vi "to string.vi"(8 "error in":errorcluster, 11 "EthernetIP configuration in":refnum<class "EthernetIP configuration.lvclass">) -> (0 "error out":errorcluster, 1 "data":string, 2 "version":string, 3 "EthernetIP configuration out":refnum<class "EthernetIP configuration.lvclass">)   [LabVIEW 2013, in "EthernetIP configuration.lvclass"]
doc: "Provides an interface for saving a module configuration to a file or other serialized data source. It is recommended that all children of this class store data in two sets--data required for its own initialization, and any data required for parent initialization--and that each implementation uses the <b>Call Parent Method</b> primitive to serialize parent information."
uses:
  EthernetIP configuration.lvclass
  <vilib>/NI/Tag Bus Module Framework/module configuration/TBM module configuration.lvclass
  EthernetIP configuration.lvclass/EthernetIP configuration.ctl
  <vilib>/NI/Tag Bus Module Framework/root configuration/unwrap data.vi
  <vilib>/NI/Tag Bus Module Framework/root configuration/TBM configuration.lvclass
  channel/EthernetIP Channel.lvclass
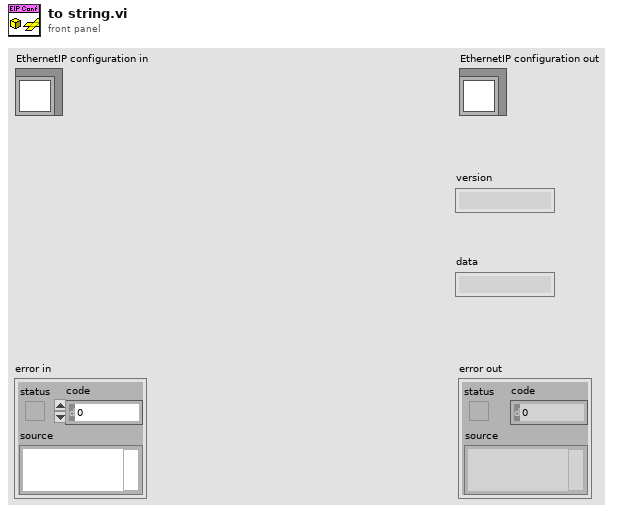
[diagram p1: front panel]
types:
  T1 = typedef "EthernetIP configuration.lvclass/assembly definition.ctl" = cluster{"name":string, "Instance ID":u32, "Type":T2, "Size (elements)":u32, "big endian?":bool, "data type":T3}
  T2 = typedef "EthernetIP configuration.lvclass/assembly type.ctl" = enum32{"Producing", "Consuming"}
  T3 = typedef "tag bus.lvlib/tag descriptor.lvclass/Data Type.ctl" = enum16{"Double", "Single", "I64", "I32", "I16", "I8", "U64", "U32", "U16", "U8", "Boolean", "String", "Array of Double", "Array of Single", "Array of I64", "Array of I32", "Array of I16", "Array of I8", "Array of U64", "Array of U32", "Array of U16", "Array of U8", "Array of Boolean", "Array of String"}
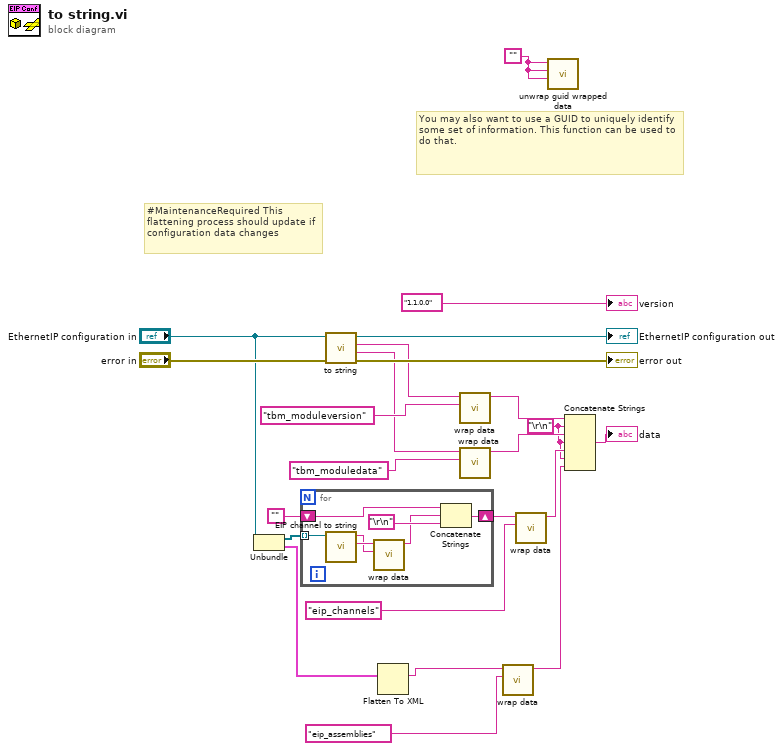
[diagram p0: block diagram]
diagram:
  w6 = "\r\n"
  w14 = ""
  # "You may also want to use a GUID to uniquely identify some set of information. This function can be used to do that."
  # "#MaintenanceRequired This flattening process should update if configuration data changes"
  n1 = Unbundle("EthernetIP configuration in") -> (w9:refnum<class "EthernetIP Channel.lvclass">[], w3:T1[])
  n2 = for {
    tunnel: w9 -> [w30] mode=indexing
    shift-right: [w26] -> w7
    shift-left: "" -> [w25]
    n3 = call "EIP channel to string.vi"("channel in"=w30) -> ("channel data"=w29:string, "identifier"=w28:string)  [unwired: 9 in]
    n4 = call <vilib>:"wrap data.vi"("identifier"=w28, "data to wrap"=w29) -> ("wrapped data"=w24:string)  [unwired: 9 in]
    n5 = Concatenate Strings(w25, w24, "\r\n") -> (w26:string)
  }
  n6 = call-parent "to string.vi"("error in"="error in", "module configuration in"="EthernetIP configuration in") -> ("error out"=→"error out":errorcluster, "data"=w15:string, "version"=w16:string, "module configuration out"=→"EthernetIP configuration out":refnum<class "EthernetIP configuration.lvclass">)  [unwired: 6 in]
  n7 = Flatten To XML(anything=w3) -> (xml string=w2:string)
  n8 = call <vilib>:"wrap data.vi"("identifier"="tbm_moduleversion" ("additional identifier"), "data to wrap"=w16) -> ("wrapped data"=w18:string)  [unwired: 9 in]
  n9 = call <vilib>:"wrap data.vi"("identifier"="tbm_moduledata" ("additional identifier"), "data to wrap"=w15) -> ("wrapped data"=w17:string)  [unwired: 9 in]
  n10 = call <vilib>:"wrap data.vi"("identifier"="eip_assemblies" ("additional identifier"), "data to wrap"=w2) -> ("wrapped data"=w4:string)  [unwired: 9 in]
  n11 = call <vilib>:"wrap data.vi"("identifier"="eip_channels" ("additional identifier"), "data to wrap"=w7) -> ("wrapped data"=w11:string)  [unwired: 9 in]
  n12 = call <vilib>:"unwrap guid wrapped data.vi"("identifier"=w14, "uuid"=w14, "data to unwrap"=w14) -> ()  [unwired: 7 in, 2 out]
  n13 = Concatenate Strings(w18, w6, w17, w6, w11, w6, w4) -> (→"data":string)
  "version" <- "1.1.0.0" ("current version")
